vi "ContinuousScanMain.vi"() -> ()   [LabVIEW 2018]
uses:
  Tektronik3102/Tecktronik action loop.ctl
  MasterStatus.ctl
  ActiveSlaves.ctl
  TargetScanControlArray.ctl
  VI_tags.ctl
  ActionSlaveVariable.ctl
  NetworkStream/NetworkStreamData.ctl
  support/Network Stream Writer.ctl
  logFileStatus.ctl
  tests/SlaveTag.ctl
  <vilib>/dex/Stream Element Allocation Mode.ctl
  NetworkStream/NetworkStream.lvlib
  MasterProgramSupportFunctions.lvlib
  <resource>/objmgr/ni.dex.rc
  MySharedVariables.lvlib
  Read and Save Files/RW_Protocols.lvlib
panel:
  out "elements":T1[](array[typedef])
  out "Nscans":i32
  in  "scan control array":T2
  out "# elements in queue 2":i32
  out "hash":u64
  out "x .or. y?":bool
  in  "Tab Control":enum32{"main", "configuration", "scan list"}(tab)
  in  "Save Button":bool
  out "done":bool
  in  "Exit":bool
  in  "launch":bool
  in  "update loop":bool
  out "N shots":i32
  out "loop in progress":u8(slide) max=6
  in  "saving folder":path=path "D:/Data/Mai/test target/logfile"
  in  "name or relative path":string
  in  "Active slaves":T5={"camera"=TRUE, "Tektronik"=TRUE, "Motors"=FALSE, "Gage"=FALSE}
  out "Table 2":string[][](table) caption="updated scan list"
  out "MasterStatusShared":T6
  in  "tektronik":enum32{"Tektronik", "Configuration"}(tab)
  out "Tecktronik contected":bool caption="Connected"
  out "Tecktronik connection status":T7
  in  "tektro wait for":T5
  in  "camera":enum32{"Ximea", "Configuration"}(tab)
  in  "ximea wait for":T5
  out "IC camera connection status":T7
  out "IC camera connected":bool caption="Connected"
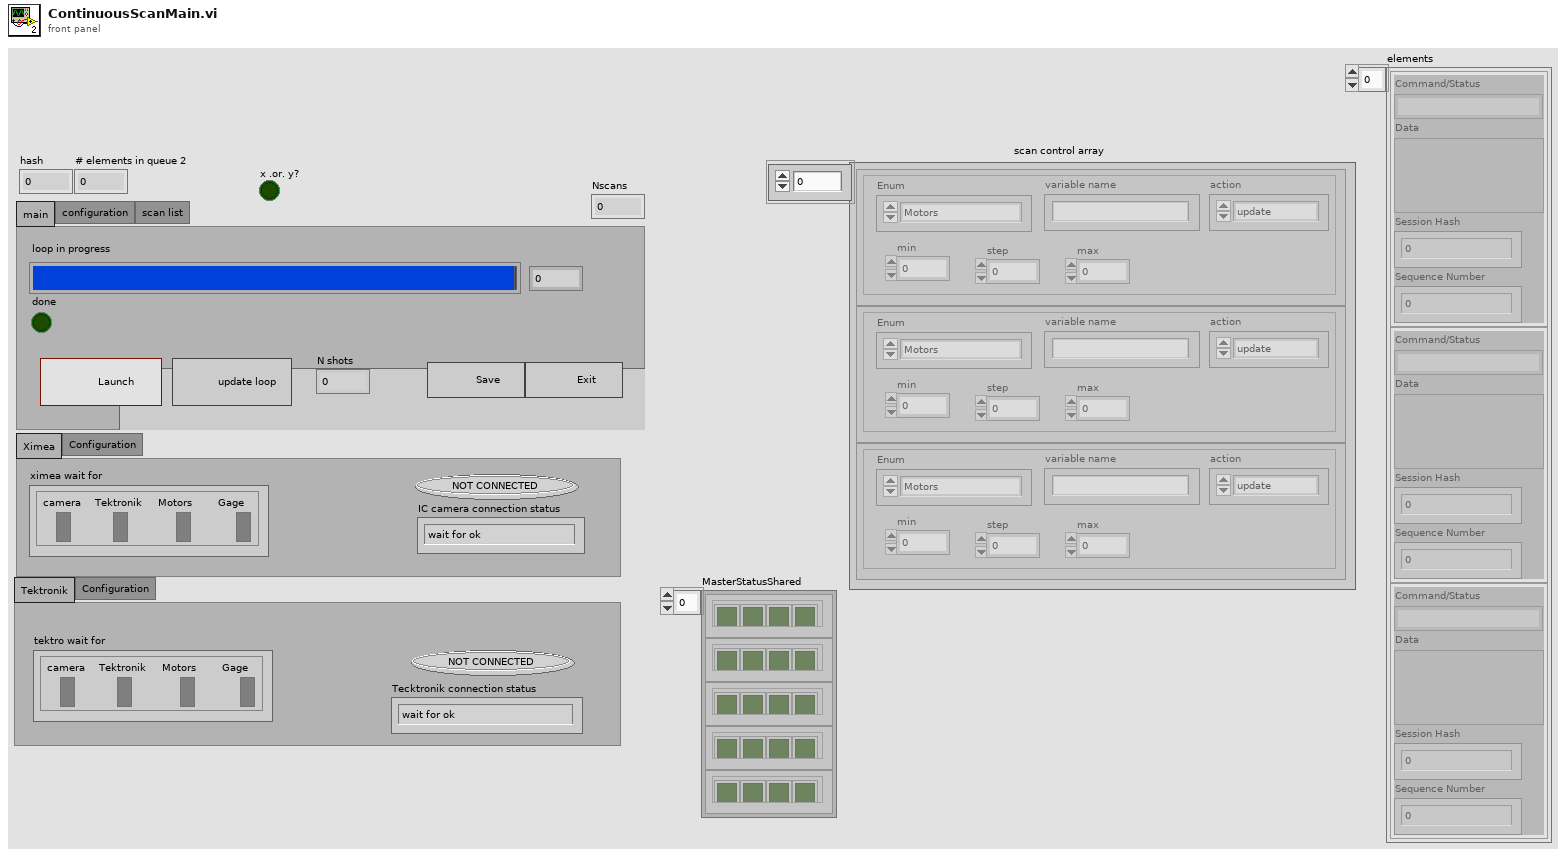
[diagram p1: front panel]
types:
  T1 = typedef "NetworkStream.lvlib/NetworkStreamData.ctl" = cluster{"Command/Status":string, "Data":variant, "Session Hash":u64, "Sequence Number":u64}
  T2 = typedef "MasterProgramSupportFunctions.lvlib/TargetScanControlArray.ctl" = cluster{"min":dbl, "step":dbl, "max":dbl, "Enum":T3, "variable name":string, "action":T4}[]
  T3 = typedef "MasterProgramSupportFunctions.lvlib/VI_tags.ctl" = enum16{"Motors", "Gage", "Tektro3107", "XimeaMainCamera", "ContinuousMainScan"}
  T4 = typedef "MasterProgramSupportFunctions.lvlib/ActionSlaveVariable.ctl" = enum16{"update", "event"}
  T5 = typedef "MasterProgramSupportFunctions.lvlib/ActiveSlaves.ctl" = cluster{"camera":bool, "Tektronik":bool, "Motors":bool, "Gage":bool}
  T6 = typedef "MySharedVariables.lvlib/MasterStatus.ctl" = cluster{"Camera done":bool, "Tektronik done":bool, "Motors done":bool, "Gage done":bool}[]
  T7 = typedef "Tecktronik action loop.ctl" = enum16{"wait for ok", "error", "ready", "write log file", "waiting for connection", "exit", "sending command"}
  T8 = typedef "logFileStatus.ctl" = enum16{"saving log", "exit", "waiting"}
  T9 = typedef "Network Stream Writer.ctl" = cluster{"Hash":u64, "writer endpoint":refnum<k21>, "Sequence Number":u64}
  T10 = typedef "SlaveTag.ctl" = enum16{"Gage", "Tektronik", "Motors", "IC camera"}
  T11 = typedef "Stream Element Allocation Mode.ctl" = u32
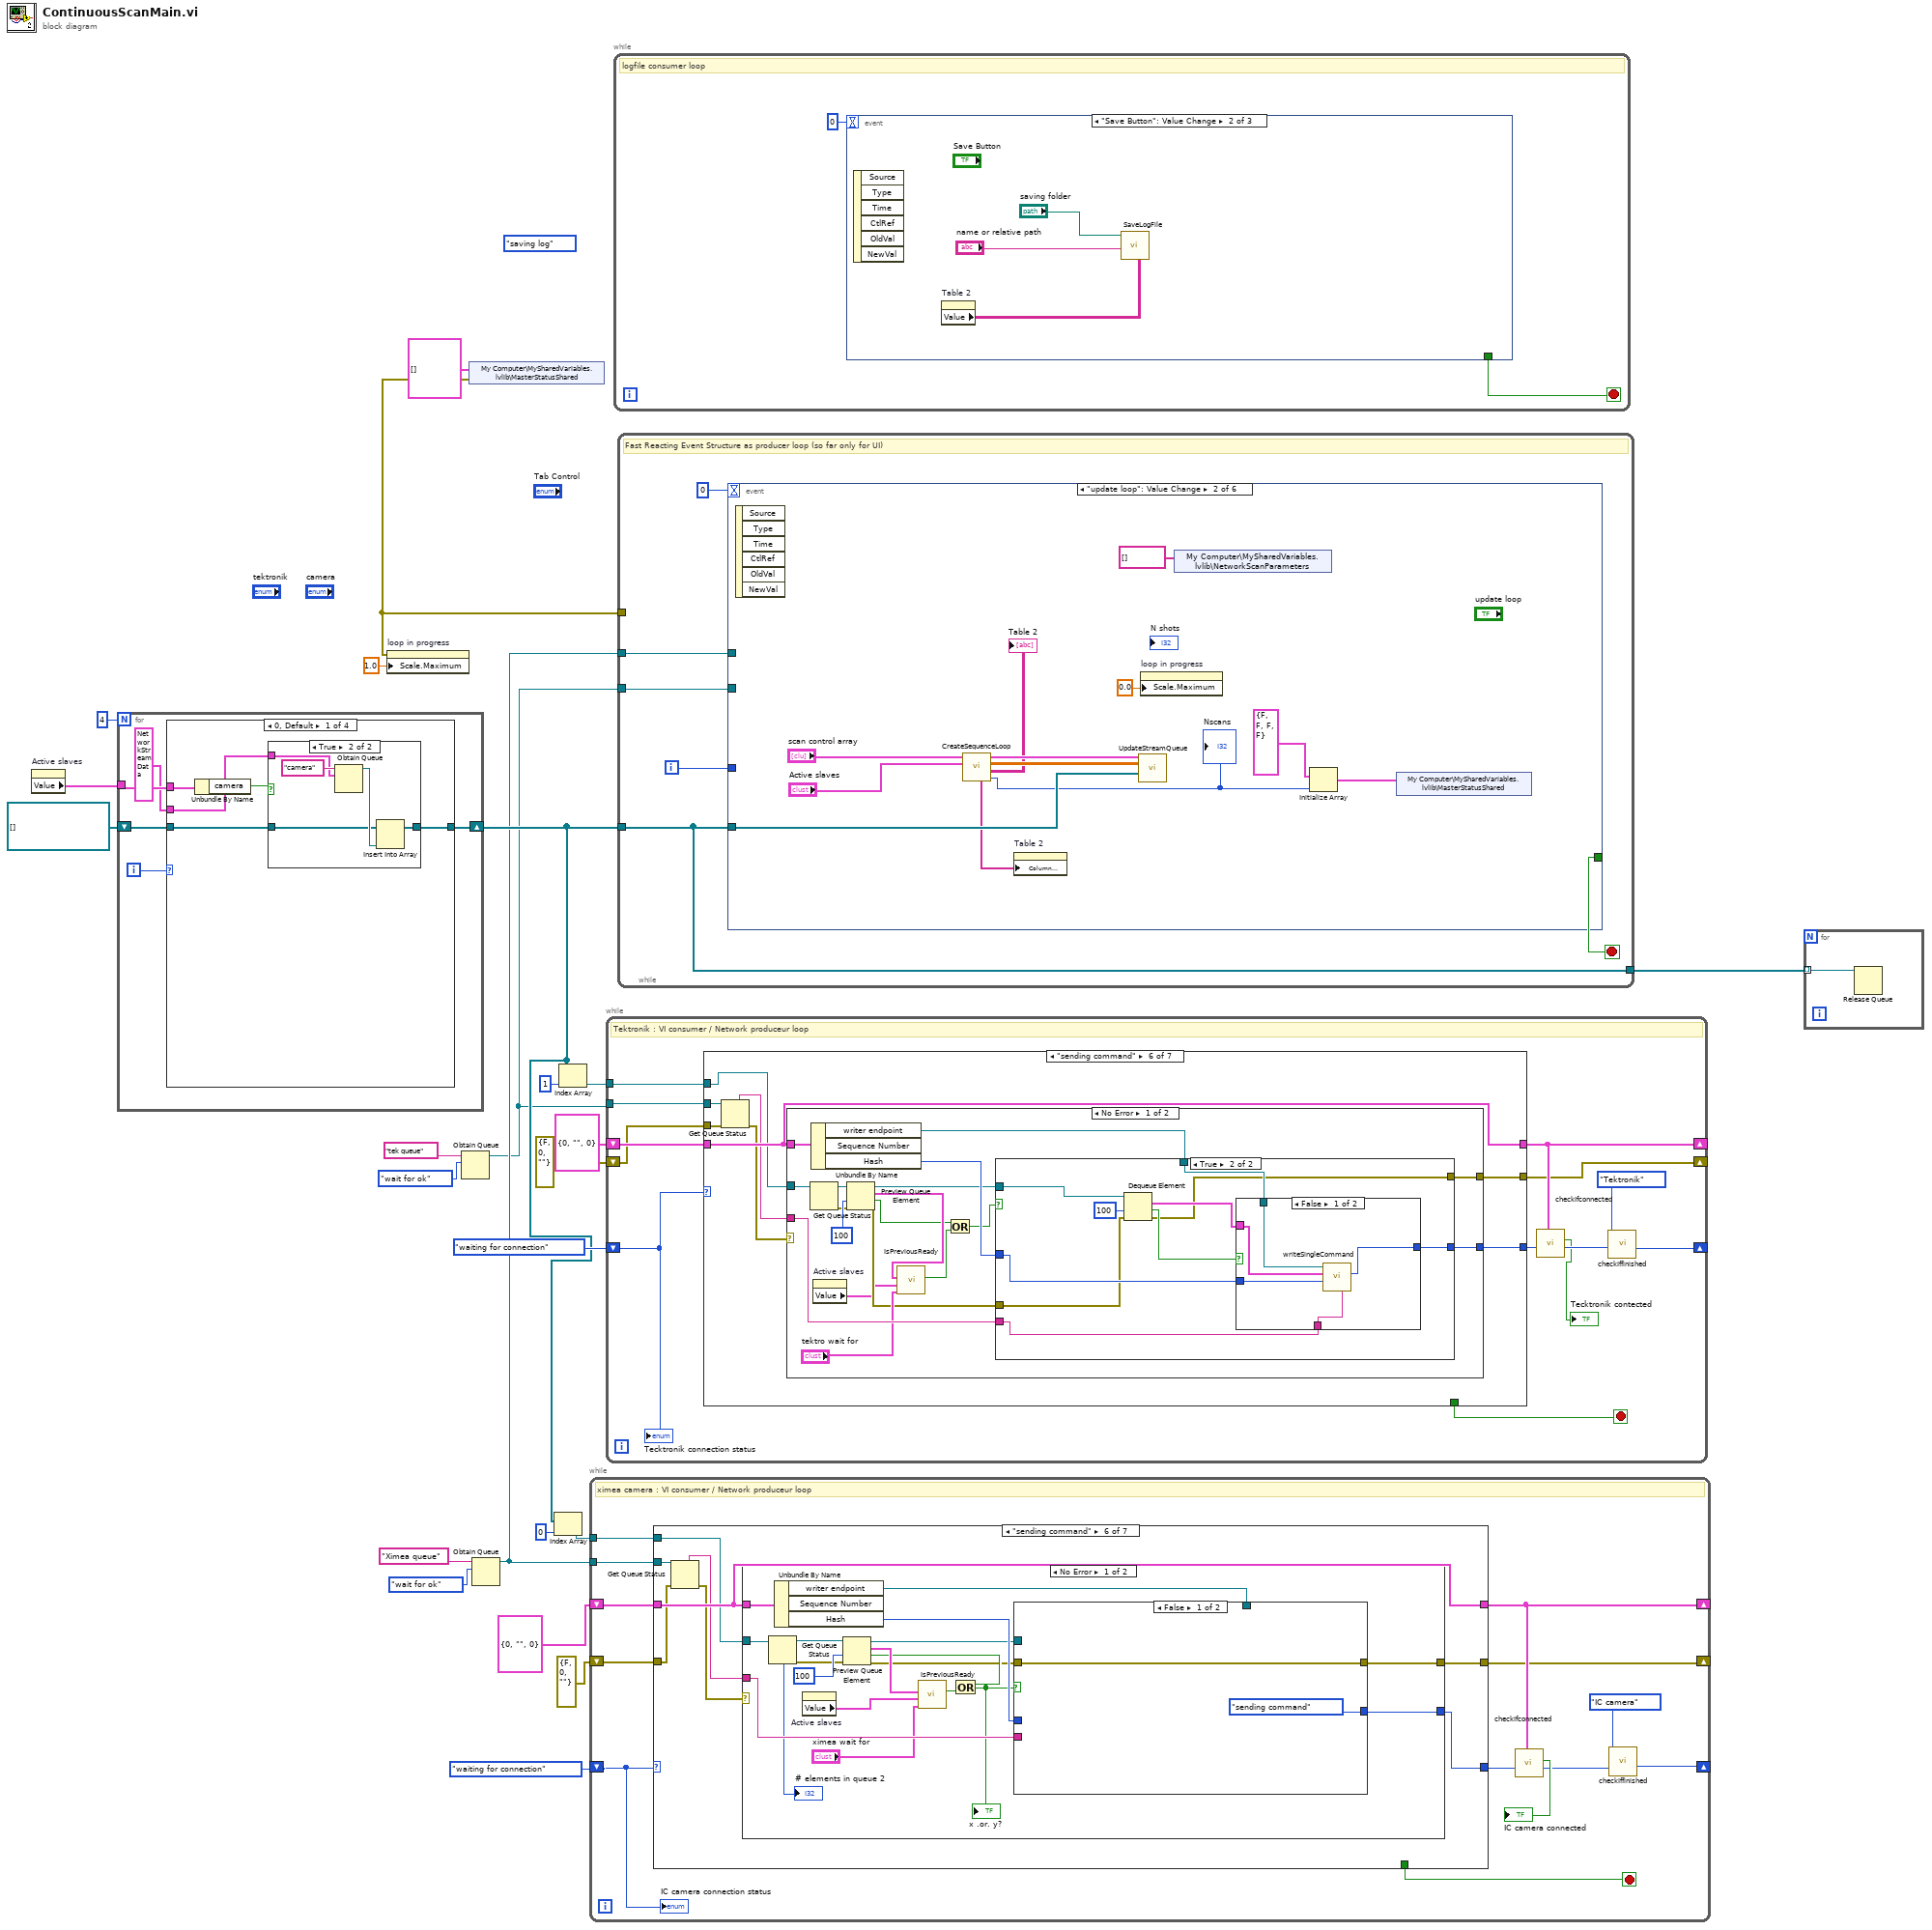
[diagram p0: block diagram]
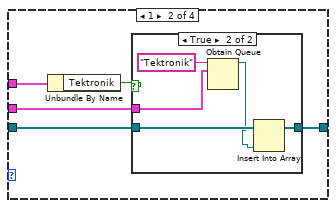
[diagram p3: hidden frame]
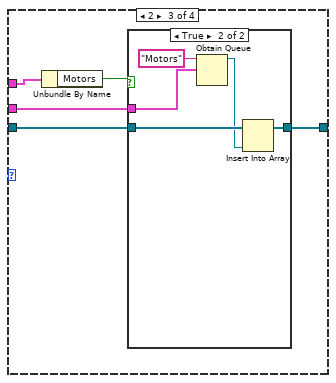
[diagram p5: hidden frame]
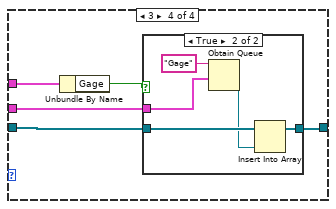
[diagram p7: hidden frame]
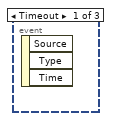
[diagram p9: hidden frame]
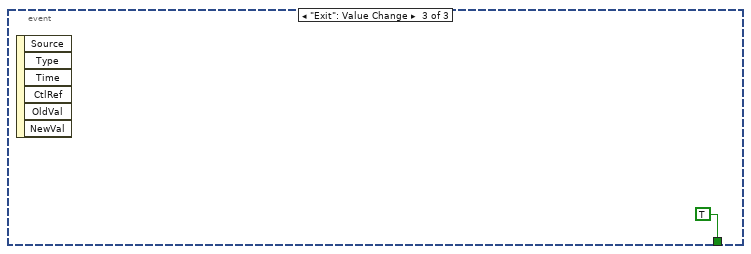
[diagram p10: hidden frame]
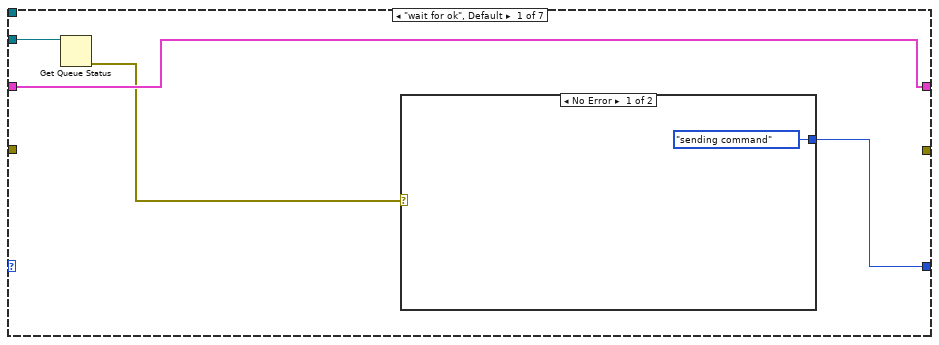
[diagram p11: hidden frame]
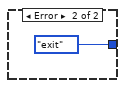
[diagram p12: hidden frame]
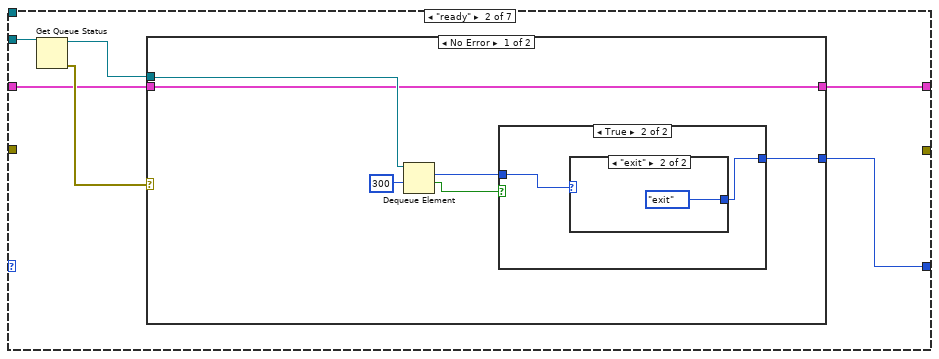
[diagram p13: hidden frame]
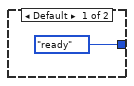
[diagram p15: hidden frame]
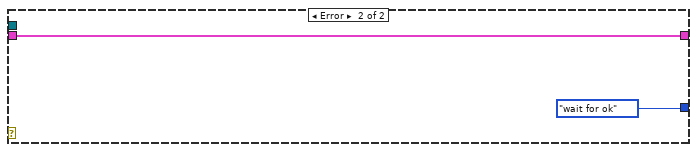
[diagram p16: hidden frame]
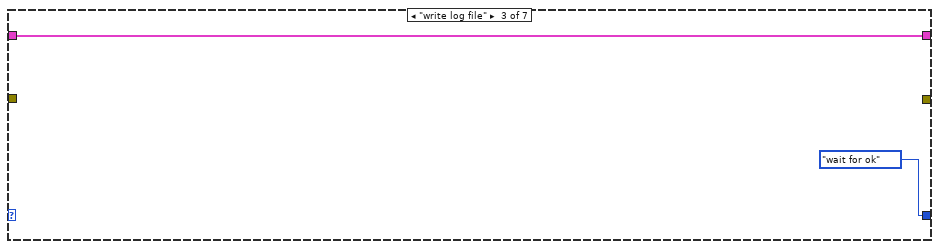
[diagram p17: hidden frame]
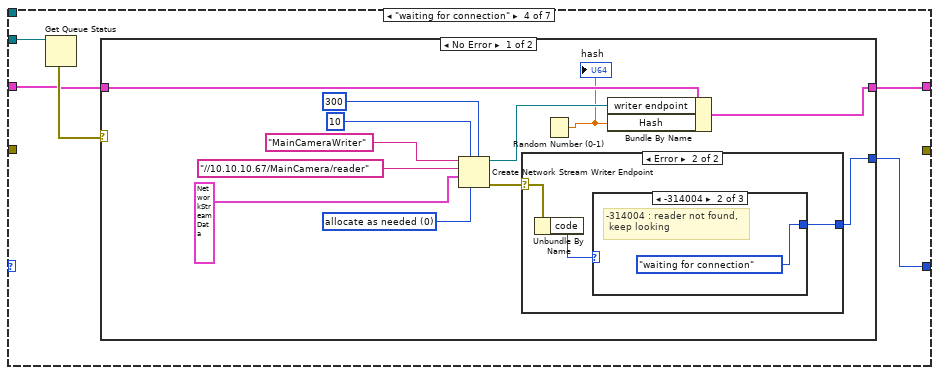
[diagram p18: hidden frame]
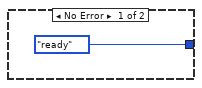
[diagram p19: hidden frame]
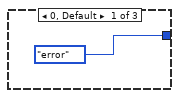
[diagram p20: hidden frame]
diagram:
  (unwired) logFileStatus."saving log" ("DeviceState")
  n1 = property on="Active slaves" class="Clust (strict)"() -> ("Value"=w14:T5)  [unwired: 2 in, 2 out]
  n2 = for {
    N: 4 -> [_]
    tunnel: w14 -> [w29]
    shift-right: [w28] -> w7
    shift-left: refnum<queue>[] [] -> [w27]
    i -> [w26]
    n3 = case shown="0, Default" w26 {
      tunnel: w29 -> [w34 w44 w53 w64]
      tunnel: [w32 w43 w54 w65] -> w28
      tunnel: w27 -> [w31 w42 w55 w66]
      tunnel: T1 {"Command/Status"="", "Data"=variant, "Session Hash"=0, "Sequence Number"=0} ("NetworkStreamCluster") -> [w30 w41 w52 w63]
      frame 0, Default {
        n4 = Unbundle By Name(w34) -> ("camera"=w33:bool)
        n5 = case shown="True" w33 {
          tunnel: [w35 w38] -> w32
          tunnel: w31 -> [w35 w37]
          tunnel: w30 -> [_ w36]
          frame False {
          }
          frame True {
            n6 = Obtain Queue(name (unnamed)="camera", element data type=w36) -> (queue out=w39:refnum<queue>)  [unwired: 3 in, 2 out]
            n7 = Insert Into Array(array=w37, new element=w39) -> (w38:refnum<queue>[])  [unwired: 1 in]
          }
        }
      }
      frame 1 {
        n8 = Unbundle By Name(w44) -> ("Tektronik"=w45:bool)
        n9 = case shown="True" w45 {
          tunnel: [w46 w50] -> w43
          tunnel: w42 -> [w46 w49]
          tunnel: w41 -> [_ w48]
          frame False {
          }
          frame True {
            n10 = Obtain Queue(name (unnamed)="Tektronik", element data type=w48) -> (queue out=w47:refnum<queue>)  [unwired: 3 in, 2 out]
            n11 = Insert Into Array(array=w49, new element=w47) -> (w50:refnum<queue>[])  [unwired: 1 in]
          }
        }
      }
      frame 2 {
        n12 = Unbundle By Name(w53) -> ("Motors"=w56:bool)
        n13 = case shown="True" w56 {
          tunnel: [w57 w61] -> w54
          tunnel: w55 -> [w57 w60]
          tunnel: w52 -> [_ w59]
          frame False {
          }
          frame True {
            n14 = Obtain Queue(name (unnamed)="Motors", element data type=w59) -> (queue out=w58:refnum<queue>)  [unwired: 3 in, 2 out]
            n15 = Insert Into Array(array=w60, new element=w58) -> (w61:refnum<queue>[])  [unwired: 1 in]
          }
        }
      }
      frame 3 {
        n16 = Unbundle By Name(w64) -> ("Gage"=w67:bool)
        n17 = case shown="True" w67 {
          tunnel: [w68 w72] -> w65
          tunnel: w66 -> [w68 w71]
          tunnel: w63 -> [_ w70]
          frame False {
          }
          frame True {
            n18 = Obtain Queue(name (unnamed)="Gage", element data type=w70) -> (queue out=w69:refnum<queue>)  [unwired: 3 in, 2 out]
            n19 = Insert Into Array(array=w71, new element=w69) -> (w72:refnum<queue>[])  [unwired: 1 in]
          }
        }
      }
    }
  }
  n20 = Obtain Queue(name (unnamed)="tek queue", element data type=Tecktronik_action_loop."wait for ok" ("DeviceState")) -> (queue out=w3:refnum<queue>)  [unwired: 3 in, 2 out]
  n21 = shared-variable "My Computer\\MySharedVariables.lvlib\\MasterStatusShared"(T6 [] ("MasterStatusShared")) -> (error out=w17:errorcluster)  [unwired: 1 in]
  n22 = property on="loop in progress" class="Slide (strict)"(error in=w17, "Scale.Maximum"=1.0 ("Scale.Range:Maximum")) -> ()  [unwired: 1 in, 2 out]
  n23 = Obtain Queue(name (unnamed)="Ximea queue", element data type=Tecktronik_action_loop."wait for ok" ("DeviceState")) -> (queue out=w4:refnum<queue>)  [unwired: 3 in, 2 out]
  n24 = Index Array(array=w7, index=0) -> (element=w5:refnum<queue>)
  n25 = Index Array(array=w7, index=1) -> (element=w10:refnum<queue>)
  n26 = while {
    shift-right: [w82] -> _
    shift-left: T9 {"Hash"=0, "writer endpoint"="", "Sequence Number"=0} ("DeviceData") -> [w83]
    shift-right: [w78] -> _
    shift-left: Tecktronik_action_loop."waiting for connection" ("DeviceState") -> [w84]
    tunnel: w4 -> [w85]
    tunnel: w5 -> [w76]
    shift-right: [w75] -> _
    shift-left: errorcluster {"status"=FALSE, "code"=0, "source"=""} ("error out") -> [w74]
    stop <- w86 stop-if-true
    # "ximea camera : VI consumer / Network produceur loop"
    n27 = case shown="\"sending command\"" w84 {
      tunnel: [_ _ _ _ TRUE _ _] -> w86
      tunnel: w83 -> [w90 w95 w113 w116 w144 w153 w194]
      tunnel: [w90 w94 w113 w115 T9 {"Hash"=0, "writer endpoint"="", "Sequence Number"=0} ("DeviceData") w153 w194] -> w82
      tunnel: w85 -> [w88 w98 _ w118 _ w152 _]
      tunnel: [w89 w93 Tecktronik_action_loop."wait for ok" ("DeviceState") w114 Tecktronik_action_loop."exit" ("DeviceState") w150 Tecktronik_action_loop."exit" ("DeviceState")] -> w81
      tunnel: w76 -> [_ _ _ _ _ w148 _]
      tunnel: [_ _ _ _ _ w147 _] -> w75
      tunnel: w74 -> [_ _ _ _ _ w146 _]
      frame "wait for ok", Default {
        n28 = Get Queue Status(queue=w88) -> (error out=w87:errorcluster)  [unwired: 2 in, 7 out]
        n29 = case shown="No Error" w87 {
          tunnel: [Tecktronik_action_loop."sending command" ("DeviceState") Tecktronik_action_loop."exit" ("DeviceState")] -> w89
          frame No Error {
          }
          frame Error {
          }
        }
      }
      frame "ready" {
        n30 = Get Queue Status(queue=w98) -> (queue out=w97:refnum<queue>, error out=w96:errorcluster)  [unwired: 2 in, 6 out]
        n31 = case shown="No Error" w96 {
          tunnel: w97 -> [w104 _]
          tunnel: w95 -> [w103 w111]
          tunnel: [w103 w111] -> w94
          tunnel: [w102 Tecktronik_action_loop."wait for ok" ("DeviceState")] -> w93
          frame No Error {
            n32 = Dequeue Element(queue=w104, timeout in ms (-1)=300) -> (element=w99:T7, timed out?=w100:bool)  [unwired: 1 in, 2 out]
            n33 = case shown="True" w100 {
              tunnel: w99 -> [w105 w106]
              tunnel: [w105 w107] -> w102
              frame False {
              }
              frame True {
                n34 = case shown="\"exit\"" w106 {
                  tunnel: [Tecktronik_action_loop."ready" ("DeviceState") Tecktronik_action_loop."exit" ("DeviceState")] -> w107
                  frame Default {
                  }
                  frame "exit" {
                  }
                }
              }
            }
          }
          frame Error {
          }
        }
      }
      frame "write log file" {
      }
      frame "waiting for connection" {
        n35 = Get Queue Status(queue=w118) -> (error out=w117:errorcluster)  [unwired: 2 in, 7 out]
        n36 = case shown="No Error" w117 {
          selector: w117 -> [_ w138]
          tunnel: [w120 Tecktronik_action_loop."exit" ("DeviceState")] -> w114
          tunnel: w116 -> [w124 w139]
          tunnel: [w122 w139] -> w115
          frame No Error {
            w127 = T11 0 items=["allocate as needed", "pre-allocate"] ("element allocation mode")
            n37 = Create Network Stream Writer Endpoint(5:300 ("timeout in ms (-1)"), 6:w127, 7:10 ("writer buffer size"), 9:T1 {"Command/Status"="", "Data"=variant, "Session Hash"=0, "Sequence Number"=0} ("NetworkStreamCluster"), 10:"//10.10.10.67/MainCamera/reader" ("reader url"), 11:"MainCameraWriter" ("writer url")) -> (0:w121:errorcluster, 3:w123:refnum<k21>)  [unwired: 1 in]
            n38 = case shown="Error" w121 {
              selector: w121 -> [_ w134]
              tunnel: [Tecktronik_action_loop."ready" ("DeviceState") w132] -> w120
              frame No Error {
              }
              frame Error {
                n39 = Unbundle By Name(w134) -> ("code"=w133:i32)
                n40 = case shown="-314004" w133 {
                  tunnel: [Tecktronik_action_loop."error" ("DeviceState") Tecktronik_action_loop."waiting for connection" ("DeviceState") Tecktronik_action_loop."waiting for connection" ("DeviceState")] -> w132
                  frame 0, Default {
                  }
                  frame -314004 {
                    # "-314004 : reader not found,\n keep looking"
                  }
                  frame -314101 {
                    # "-314004 : reader not found,\nafter deconnection"
                  }
                }
              }
            }
            n41 = Random Number (0-1)() -> (number: 0 to 1=w119:dbl)
            "hash" <- w119
            n42 = Bundle By Name(cluster=w124, "writer endpoint"=w123, "Hash"=w119) -> (w122:T9)
          }
          frame Error {
            # "error occurs when Queue is destroyed, meaning VI is closing"
            n43 = Unbundle By Name(w138) -> ()  [unwired: 1 out]
          }
        }
      }
      frame "exit" {
        n44 = Unbundle By Name(w144) -> ("writer endpoint"=w143:refnum<k21>)
        n45 = Destroy Stream Endpoint(11:w143) -> ()  [unwired: 1 in, 1 out]
      }
      frame "sending command" {
        n46 = Get Queue Status(queue=w152, error in (no error)=w146) -> (queue name=w149:string, error out=w151:errorcluster)  [unwired: 1 in, 6 out]
        n47 = case shown="No Error" w151 {
          selector: w151 -> [_ w191]
          tunnel: w153 -> [w170 _]
          tunnel: [w169 Tecktronik_action_loop."exit" ("DeviceState")] -> w150
          tunnel: w149 -> [w168 _]
          tunnel: w148 -> [w161 _]
          tunnel: [w155 w191] -> w147
          frame No Error {
            n48 = Get Queue Status(queue=w161) -> (queue out=w160:refnum<queue>, error out=w157:errorcluster, # elements in queue=→"# elements in queue 2":i32)  [unwired: 2 in, 5 out]
            n49 = Unbundle By Name(w170) -> ("writer endpoint"=w172:refnum<k21>, "Hash"=w171:u64)  [unwired: 1 out]
            n50 = property on="Active slaves" class="Clust (strict)"() -> ("Value"=w158:T5)  [unwired: 2 in, 2 out]
            n51 = Preview Queue Element(queue=w160, timeout in ms (-1)=100, error in (no error)=w157) -> (queue out=w166:refnum<queue>, element=w165:T1, timed out?=w163:bool, error out=w156:errorcluster)
            n52 = call "IsPreviousReady.vi"("wait for"="ximea wait for", "Active slaves"=w158, "element"=w165) -> ("is ready"=w164:bool)  [unwired: 8 in]
            n53 = Or(x=w163, y=w164) -> (x .or. y?=w162:bool)
            "x .or. y?" <- w162
            n54 = case shown="False" w162 {
              tunnel: w172 -> [_ w184]
              tunnel: w171 -> [_ w183]
              tunnel: [Tecktronik_action_loop."sending command" ("DeviceState") w180] -> w169
              tunnel: w168 -> [_ w178]
              tunnel: w166 -> [_ w177]
              tunnel: w156 -> [w173 w176]
              tunnel: [w173 w175] -> w155
              frame False {
              }
              frame True {
                n55 = Dequeue Element(queue=w177, timeout in ms (-1)=100, error in (no error)=w176) -> (element=w182:T1, timed out?=w179:bool, error out=w175:errorcluster)  [unwired: 1 out]
                n56 = case shown="False" w179 {
                  tunnel: w184 -> [w185 _]
                  tunnel: w183 -> [w189 _]
                  tunnel: w182 -> [w188 _]
                  tunnel: [w187 Tecktronik_action_loop."sending command" ("DeviceState")] -> w180
                  tunnel: w178 -> [w186 _]
                  frame False {
                    n57 = call "writeSingleCommand.vi"("String"=w186, "Session Hash"=w189, "NetworkStreamCluster"=w188, "endpoint input"=w185) -> ("next move"=w187:T7)  [unwired: 6 in, 1 out]
                  }
                  frame True {
                  }
                }
              }
            }
          }
          frame Error {
          }
        }
      }
      frame "error" {
      }
    }
    n58 = call "checkIfconnected.vi"("input stream cluster"=w82, "Input device state"=w81) -> ("NextDeviceState"=w79:T7, "Connected"=→"IC camera connected":bool)  [unwired: 7 in, 1 out]
    n59 = call "checkIffinished.vi"("InDeviceState"=w79, "Slave tag"=SlaveTag."IC camera") -> ("OutDeviceState"=w78:T7)  [unwired: 9 in]
    "IC camera connection status" <- w84
  }
  n60 = while {
    shift-right: [w204] -> _
    shift-left: T9 {"Hash"=0, "writer endpoint"="", "Sequence Number"=0} ("DeviceData") -> [w205]
    shift-right: [w201] -> _
    shift-left: Tecktronik_action_loop."waiting for connection" ("DeviceState") -> [w207]
    tunnel: w10 -> [w198]
    tunnel: w3 -> [w197]
    shift-right: [w196] -> _
    shift-left: errorcluster {"status"=FALSE, "code"=0, "source"=""} ("error out") -> [w195]
    stop <- w206 stop-if-true
    # "Tektronik : VI consumer / Network produceur loop"
    n61 = case shown="\"sending command\"" w207 {
      tunnel: [_ _ _ _ TRUE _ _] -> w206
      tunnel: w205 -> [w209 w212 w232 w235 w261 w271 w310]
      tunnel: [w209 w211 w232 w234 T9 {"Hash"=0, "writer endpoint"="", "Sequence Number"=0} ("DeviceData") w271 w310] -> w204
      tunnel: [Tecktronik_action_loop."sending command" ("DeviceState") w215 Tecktronik_action_loop."wait for ok" ("DeviceState") w236 Tecktronik_action_loop."exit" ("DeviceState") w270 Tecktronik_action_loop."exit" ("DeviceState")] -> w203
      tunnel: w198 -> [_ _ _ _ _ w267 _]
      tunnel: w197 -> [_ w210 _ w233 _ w266 _]
      tunnel: [_ _ _ _ _ w265 _] -> w196
      tunnel: w195 -> [_ _ _ _ _ w264 _]
      frame "wait for ok", Default {
      }
      frame "ready" {
        n62 = Get Queue Status(queue=w210) -> (queue out=w214:refnum<queue>, error out=w213:errorcluster)  [unwired: 2 in, 6 out]
        n63 = case shown="No Error" w213 {
          tunnel: [w221 Tecktronik_action_loop."exit" ("DeviceState")] -> w215
          tunnel: w214 -> [w219 _]
          tunnel: w212 -> [w217 w229]
          tunnel: [w217 w229] -> w211
          frame No Error {
            n64 = Unbundle By Name(w217) -> ("writer endpoint"=w218:refnum<k21>)
            n65 = property class="Network Stream Endpoint"(reference=w218) -> ("Connected"=w216:bool)  [unwired: 1 in, 2 out]
            n66 = property on="Tecktronik contected" class="Bool (strict)"("Val(Sgnl)"=w216) -> ()  [unwired: 2 in, 2 out]
            n67 = Dequeue Element(queue=w219, timeout in ms (-1)=300) -> (element=w220:T7, timed out?=w222:bool)  [unwired: 1 in, 2 out]
            n68 = case shown="True" w222 {
              tunnel: [w224 w226] -> w221
              tunnel: w220 -> [w224 w225]
              frame False {
              }
              frame True {
                n69 = case shown="Default" w225 {
                  tunnel: [Tecktronik_action_loop."ready" ("DeviceState") Tecktronik_action_loop."exit" ("DeviceState")] -> w226
                  frame Default {
                  }
                  frame "exit" {
                  }
                }
              }
            }
          }
          frame Error {
          }
        }
      }
      frame "write log file" {
      }
      frame "waiting for connection" {
        n70 = Get Queue Status(queue=w233) -> (error out=w237:errorcluster)  [unwired: 2 in, 7 out]
        n71 = case shown="No Error" w237 {
          selector: w237 -> [_ w256]
          tunnel: [w238 Tecktronik_action_loop."exit" ("DeviceState")] -> w236
          tunnel: w235 -> [w242 w257]
          tunnel: [w240 w257] -> w234
          frame No Error {
            w245 = T11 0 items=["allocate as needed", "pre-allocate"] ("element allocation mode")
            n72 = Create Network Stream Writer Endpoint(5:300 ("timeout in ms (-1)"), 6:w245, 7:10 ("writer buffer size"), 9:T1 {"Command/Status"="", "Data"=variant, "Session Hash"=0, "Sequence Number"=0} ("NetworkStreamCluster"), 10:"//10.20.20.100/Tek3102/reader" ("reader url"), 11:"Tek3102Writer" ("writer url")) -> (0:w239:errorcluster, 3:w241:refnum<k21>)  [unwired: 1 in]
            n73 = case shown="Error" w239 {
              selector: w239 -> [_ w252]
              tunnel: [Tecktronik_action_loop."ready" ("DeviceState") w250] -> w238
              frame No Error {
              }
              frame Error {
                n74 = Unbundle By Name(w252) -> ("code"=w251:i32)
                n75 = case shown="-314004" w251 {
                  tunnel: [Tecktronik_action_loop."error" ("DeviceState") Tecktronik_action_loop."waiting for connection" ("DeviceState") Tecktronik_action_loop."waiting for connection" ("DeviceState")] -> w250
                  frame 0, Default {
                  }
                  frame -314004 {
                    # "-314004 : reader not found,\n keep looking"
                  }
                  frame -314101 {
                    # "-314004 : reader not found,\nafter deconnection"
                  }
                }
              }
            }
            n76 = Bundle By Name(cluster=w242, "writer endpoint"=w241) -> (w240:T9)
          }
          frame Error {
            # "error occurs when Queue is destroyed, meaning VI is closing"
            n77 = Unbundle By Name(w256) -> ()  [unwired: 1 out]
          }
        }
      }
      frame "exit" {
        n78 = Unbundle By Name(w261) -> ("writer endpoint"=w260:refnum<k21>)
        n79 = Destroy Stream Endpoint(11:w260) -> ()  [unwired: 1 in, 1 out]
      }
      frame "sending command" {
        n80 = Get Queue Status(queue=w266, error in (no error)=w264) -> (queue name=w268:string, error out=w269:errorcluster)  [unwired: 1 in, 6 out]
        n81 = case shown="No Error" w269 {
          tunnel: w271 -> [w287 _]
          tunnel: [w286 Tecktronik_action_loop."exit" ("DeviceState")] -> w270
          tunnel: w268 -> [w285 _]
          tunnel: w267 -> [w277 _]
          tunnel: [w273 _] -> w265
          frame No Error {
            n82 = Get Queue Status(queue=w277) -> (queue out=w278:refnum<queue>, error out=w275:errorcluster)  [unwired: 2 in, 6 out]
            n83 = Unbundle By Name(w287) -> ("writer endpoint"=w289:refnum<k21>, "Hash"=w288:u64)  [unwired: 1 out]
            n84 = property on="Active slaves" class="Clust (strict)"() -> ("Value"=w272:T5)  [unwired: 2 in, 2 out]
            n85 = Preview Queue Element(queue=w278, timeout in ms (-1)=100, error in (no error)=w275) -> (queue out=w279:refnum<queue>, element=w283:T1, timed out?=w282:bool, error out=w274:errorcluster)
            n86 = call "IsPreviousReady.vi"("wait for"="tektro wait for", "Active slaves"=w272, "element"=w283) -> ("is ready"=w281:bool)  [unwired: 8 in]
            n87 = Or(x=w282, y=w281) -> (x .or. y?=w280:bool)
            n88 = case shown="True" w280 {
              tunnel: w289 -> [_ w296]
              tunnel: w288 -> [_ w295]
              tunnel: [Tecktronik_action_loop."sending command" ("DeviceState") w301] -> w286
              tunnel: w285 -> [_ w297]
              tunnel: w279 -> [_ w299]
              tunnel: w274 -> [w290 w293]
              tunnel: [w290 w292] -> w273
              frame False {
              }
              frame True {
                n89 = Dequeue Element(queue=w299, timeout in ms (-1)=100, error in (no error)=w293) -> (element=w294:T1, timed out?=w298:bool, error out=w292:errorcluster)  [unwired: 1 out]
                n90 = case shown="False" w298 {
                  tunnel: [w306 Tecktronik_action_loop."sending command" ("DeviceState")] -> w301
                  tunnel: w297 -> [w305 _]
                  tunnel: w296 -> [w304 _]
                  tunnel: w295 -> [w303 _]
                  tunnel: w294 -> [w302 _]
                  frame False {
                    n91 = call "writeSingleCommand.vi"("String"=w305, "Session Hash"=w303, "NetworkStreamCluster"=w302, "endpoint input"=w304) -> ("next move"=w306:T7)  [unwired: 6 in, 1 out]
                  }
                  frame True {
                  }
                }
              }
            }
          }
          frame Error {
          }
        }
      }
      frame "error" {
      }
    }
    n92 = call "checkIfconnected.vi"("input stream cluster"=w204, "Input device state"=w203) -> ("NextDeviceState"=w202:T7, "Connected"=→"Tecktronik contected":bool)  [unwired: 7 in, 1 out]
    n93 = call "checkIffinished.vi"("InDeviceState"=w202, "Slave tag"=SlaveTag."Tektronik") -> ("OutDeviceState"=w201:T7)  [unwired: 9 in]
    "Tecktronik connection status" <- w207
  }
  n94 = while {
    stop <- w311 stop-if-true
    # "logfile consumer loop"
    n95 = event shown="[1] \"Save Button\": Value Change" {
      selector: _ -> [_ _ _]
      dyn-events: _ -> [_ _ _]
      timeout: 0 -> [_ _ _]
      tunnel: [_ _ TRUE] -> w311
      event Timeout {
        n96 = event-data() -> ()  [unwired: 1 in, 3 out]
      }
      event "Save Button": Value Change {
        n97 = event-data() -> ()  [unwired: 1 in, 6 out]
        n98 = property on="Table 2" class="Tbl (strict)"() -> ("Value"=w313:string[][])  [unwired: 2 in, 2 out]
        n99 = call "SaveLogFile.vi"("logs in"=w313, "name or relative path"="name or relative path", "saving folder"="saving folder") -> ()  [unwired: 8 in, 1 out]
      }
      event "Exit": Value Change {
        n100 = event-data() -> ()  [unwired: 1 in, 6 out]
      }
    }
  }
  n101 = while {
    tunnel: w4 -> [w320]
    tunnel: w17 -> [_]
    tunnel: w7 -> [w318]
    tunnel: [w318] -> w13
    tunnel: w3 -> [w317]
    i -> [w319]
    stop <- w321 stop-if-true
    # "Fast Reacting Event Structure as producer loop (so far only for UI)"
    n102 = event shown="[1] \"update loop\": Value Change" {
      selector: _ -> [_ _ _ _ _ _]
      dyn-events: _ -> [_ _ _ _ _ _]
      timeout: 0 -> [_ _ _ _ _ _]
      tunnel: [_ _ _ TRUE _ _] -> w321
      tunnel: w320 -> [_ _ w346 w349 _ w360]
      tunnel: w319 -> [_ _ _ _ _ _]
      tunnel: w318 -> [w327 w337 _ _ _ _]
      tunnel: w317 -> [_ _ w343 w347 w356 _]
      event Timeout {
        n103 = event-data() -> ()  [unwired: 1 in, 3 out]
        n104 = call "ReadMasterStatus.vi"() -> ("done"=→"done":bool, "loop in progress"=→"loop in progress":u8)  [unwired: 10 in]
        n105 = Index Array(array=w327, index=0) -> (element=w325:refnum<queue>)
        n106 = shared-variable "My Computer\\MySharedVariables.lvlib\\MasterStatusShared"() -> (→"MasterStatusShared":T6)  [unwired: 1 in, 1 out]
        n107 = Get Queue Status(queue=w325, return elements? (F)=TRUE) -> (elements=→"elements":T1[])  [unwired: 1 in, 7 out]
      }
      event "update loop": Value Change {
        n108 = event-data() -> ()  [unwired: 1 in, 6 out]
        n109 = call "CreateSequenceLoop.vi"("Active slaves"="Active slaves", "scan control array"="scan control array") -> ("Nscans"=w333:i32, "Table 2"=→"Table 2":string[][], "output array"=w338:dbl[][], "scan header array"=w339:cluster{"Enum":T3, "variable name":string}[], "header"=w334:string[])  [unwired: 5 in]
        "Nscans" <- w333
        n110 = property on="Table 2" class="Tbl (strict)"("Column Headers[]"=w334) -> ()  [unwired: 2 in, 2 out]
        n111 = call "UpdateStreamQueue.vi"("scan header array"=w339, "output array"=w338, "Array"=w337) -> ()  [unwired: 8 in]
        n112 = property on="loop in progress" class="Slide (strict)"("Scale.Maximum"=0.0 ("Scale.Range:Maximum")) -> ()  [unwired: 2 in, 2 out]
        n113 = shared-variable "My Computer\\MySharedVariables.lvlib\\NetworkScanParameters"(string[] [] ("NetworkScanParameters")) -> ()  [unwired: 1 in, 1 out]
        n114 = Initialize Array(cluster{bool, bool, bool, bool} {FALSE, FALSE, FALSE, FALSE}, w333) -> (w331:cluster{bool, bool, bool, bool}[])
        n115 = shared-variable "My Computer\\MySharedVariables.lvlib\\MasterStatusShared"(w331) -> ()  [unwired: 1 in, 1 out]
      }
      event "launch": Value Change {
        n116 = event-data() -> ()  [unwired: 1 in, 6 out]
        n117 = Enqueue Element(queue=w343, element=Tecktronik_action_loop."sending command") -> ()  [unwired: 2 in, 3 out]
        n118 = Enqueue Element(queue=w346, element=Tecktronik_action_loop."sending command") -> ()  [unwired: 2 in, 3 out]
      }
      event "Exit": Value Change {
        n119 = event-data() -> ()  [unwired: 1 in, 6 out]
        n120 = Enqueue Element At Opposite End(queue=w347, element=Tecktronik_action_loop."exit") -> (queue out=w354:refnum<queue>, error out=w352:errorcluster)  [unwired: 2 in, 1 out]
        n121 = Enqueue Element At Opposite End(queue=w349, element=Tecktronik_action_loop."exit") -> (queue out=w351:refnum<queue>, error out=w350:errorcluster)  [unwired: 2 in, 1 out]
        n122 = Release Queue(queue=w354, error in (no error)=w352) -> ()  [unwired: 1 in, 3 out]
        n123 = Release Queue(queue=w351, error in (no error)=w350) -> ()  [unwired: 1 in, 3 out]
      }
      event "Tecktronik contected": Value Change {
        n124 = event-data() -> ("NewVal"=w357:bool)  [unwired: 1 in, 5 out]
        n125 = case shown="False" w357 {
          tunnel: w356 -> [w358 _]
          frame False {
            n126 = Enqueue Element At Opposite End(queue=w358, element=Tecktronik_action_loop."waiting for connection") -> ()  [unwired: 2 in, 3 out]
          }
          frame True {
          }
        }
      }
      event "IC camera connected": Value Change {
        n127 = event-data() -> ("NewVal"=w361:bool)  [unwired: 1 in, 5 out]
        n128 = case shown="False" w361 {
          tunnel: w360 -> [w363 _]
          frame False {
            n129 = Enqueue Element At Opposite End(queue=w363, element=Tecktronik_action_loop."waiting for connection") -> ()  [unwired: 2 in, 3 out]
          }
          frame True {
          }
        }
      }
    }
  }
  n130 = for {
    tunnel: w13 -> [w364] mode=indexing
    n131 = Release Queue(queue=w364) -> ()  [unwired: 2 in, 3 out]
  }
